vi "read_sample_weight.vi"(8 "error in (no error)":errorcluster, 11 "TheilSenRegressor in":refnum<class "TheilSenRegressor.lvclass">) -> (0 "error out":errorcluster, 2 "sample_weight":dbl[](array[numeric]), 3 "TheilSenRegressor out":refnum<class "TheilSenRegressor.lvclass">)   [LabVIEW 2020, in "TheilSenRegressor.lvclass"]
uses:
  TheilSenRegressor.lvclass
  TheilSenRegressor.lvclass/TheilSenRegressor.ctl
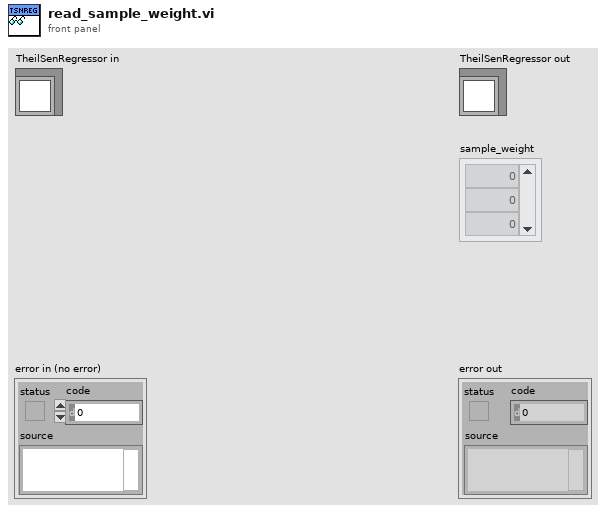
[diagram p1: front panel]
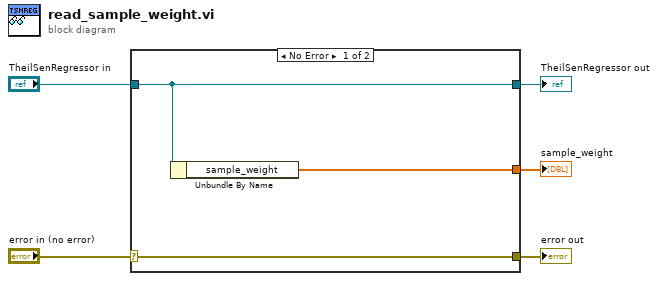
[diagram p0: block diagram]
diagram:
  n1 = case shown="No Error" "error in (no error)" {
    selector: "error in (no error)" -> [w8 w9]
    tunnel: [w8 w9] -> w4
    tunnel: [w7 w10] -> w2
    tunnel: "TheilSenRegressor in" -> [w7 w10]
    tunnel: [w6 _] -> w1
    frame No Error {
      n2 = Unbundle By Name(w7) -> ("sample_weight"=w6:dbl[])
    }
    frame Error {
    }
  }
  "error out" <- w4
  "TheilSenRegressor out" <- w2
  "sample_weight" <- w1
